vi "Update_Best_Positions.vi"(0 "Target Value":dbl, 1 "Global Best Residual":dbl, 2 "Global Best Position":dbl, 5 "Particle Best Position":dbl[](array[numeric]), 7 "Particle Best Residual":dbl[](array[numeric]), 9 "Current Partical Value":dbl[](array[numeric]), 11 "Current Particle Position":dbl[](array[numeric])) -> (4 "Updated Best Particle Residual":dbl[](array[numeric]), 6 "Updated Particle Best Position":dbl[](array[numeric]), 8 "Current Partical Value Out":dbl[](array[numeric]), 10 "Current Particle Position Out":dbl[](array[numeric]), 13 "Updated Global Best Residual":dbl, 14 "Updated Global Best Position":dbl)   [LabVIEW 2011]
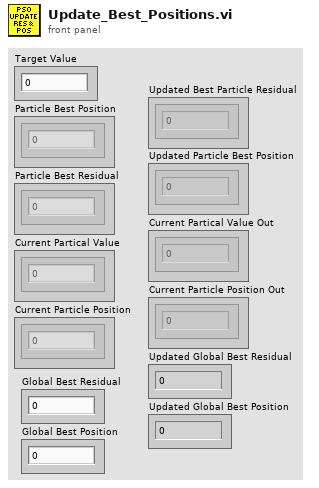
[diagram p1: front panel]
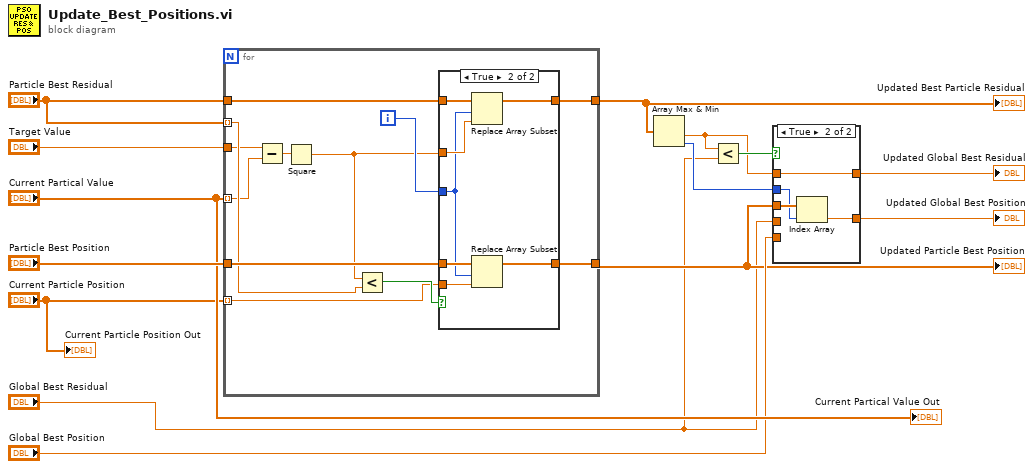
[diagram p0: block diagram]
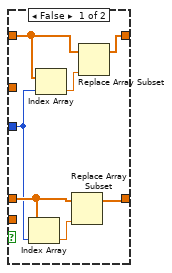
[diagram p3: hidden frame]
diagram:
  n1 = for {
    tunnel: "Particle Best Position" -> [w23]
    tunnel: "Target Value" -> [w18]
    tunnel: "Current Partical Value" -> [w17] mode=indexing
    tunnel: "Particle Best Residual" -> [w25]
    tunnel: "Current Particle Position" -> [w22] mode=indexing
    tunnel: [w21] -> w7
    tunnel: [w20] -> w10
    tunnel: "Particle Best Residual" -> [w19] mode=indexing
    i -> [w24]
    n2 = Subtract(x=w18, y=w17) -> (x-y=w16:dbl)
    n3 = Square(x=w16) -> (x^2=w15:dbl)
    n4 = Less?(x=w15, y=w19) -> (x < y?=w26:bool)
    n5 = case shown="True" w26 {
      tunnel: w25 -> [w28 w40]
      tunnel: w15 -> [_ w39]
      tunnel: w24 -> [w27 w37]
      tunnel: w23 -> [w32 w38]
      tunnel: w22 -> [_ w36]
      tunnel: [w31 w35] -> w21
      tunnel: [w29 w34] -> w20
      frame False {
        n6 = Index Array(array=w32, index=w27) -> (element=w33:dbl)
        n7 = Index Array(array=w28, index=w27) -> (element=w30:dbl)
        n8 = Replace Array Subset(array=w32, new element=w33) -> (w31:dbl[])  [unwired: 1 in]
        n9 = Replace Array Subset(array=w28, new element=w30) -> (w29:dbl[])  [unwired: 1 in]
      }
      frame True {
        n10 = Replace Array Subset(array=w40, new element=w39, index=w37) -> (w34:dbl[])
        n11 = Replace Array Subset(array=w38, new element=w36, index=w37) -> (w35:dbl[])
      }
    }
  }
  "Updated Best Particle Residual" <- w10
  "Updated Particle Best Position" <- w7
  n12 = Array Max & Min(array=w10) -> (min value=w2:dbl, min index (indices)=w6:i32)  [unwired: 2 out]
  n13 = Less?(x=w2, y="Global Best Residual") -> (x < y?=w9:bool)
  n14 = case shown="True" w9 {
    tunnel: "Global Best Position" -> [w42 _]
    tunnel: w7 -> [_ w46]
    tunnel: w6 -> [_ w45]
    tunnel: w2 -> [_ w43]
    tunnel: "Global Best Residual" -> [w41 _]
    tunnel: [w42 w44] -> w5
    tunnel: [w41 w43] -> w4
    frame False {
    }
    frame True {
      n15 = Index Array(array=w46, index=w45) -> (element=w44:dbl)
    }
  }
  "Updated Global Best Position" <- w5
  "Updated Global Best Residual" <- w4
  "Current Partical Value Out" <- "Current Partical Value"
  "Current Particle Position Out" <- "Current Particle Position"
